vi "Initialize.vi"(8 "error in (no error)":errorcluster, 11 "Test 1 in":refnum<class "Test Caller.lvclass">) -> (0 "error out":errorcluster, 3 "Test 1 out":refnum<class "Test Caller.lvclass">)   [LabVIEW 2020, in "Scratchpad.lvlib" / "Test Caller.lvlib" / "Test Caller.lvclass"]
uses:
  Test Caller.lvclass
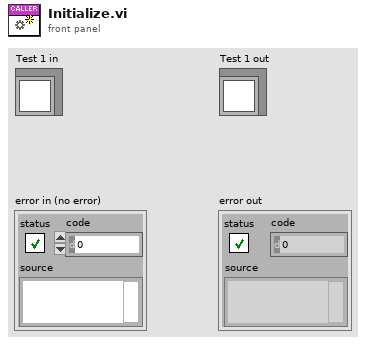
[diagram p1: front panel]
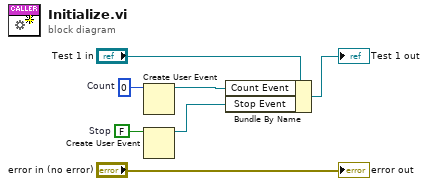
[diagram p0: block diagram]
diagram:
  w2 = FALSE  # Stop
  w4 = 0  # Count
  n1 = Create User Event(user event datatype=w4) -> (user event=w3:refnum<user-event>)  [unwired: 1 in, 1 out]
  n2 = Create User Event(user event datatype=w2) -> (user event=w1:refnum<user-event>)  [unwired: 1 in, 1 out]
  n3 = Bundle By Name(cluster="Test 1 in", "Count Event"=w3, "Stop Event"=w1) -> (→"Test 1 out":refnum<class "Test Caller.lvclass">)
  "error out" <- "error in (no error)"
